vi "Parse Field Type.vi"(6 "Field in":T1={"Name"="", "Number"=0, "Optional"=FALSE, "Repeated"=FALSE, "Type"={"Type"=enum."double", "Subtype"=""}, "Key Type"={"Type"=enum."double", "Subtype"=""}, "Value Type"={"Type"=enum."double", "Subtype"=""}}, 8 "error in (no error)":errorcluster, 10 "Text":string, 11 "ProtoParser in":refnum<class "ProtoParser.lvclass">) -> (0 "error out":errorcluster, 2 "Remaining":string, 3 "ProtoParser out":refnum<class "ProtoParser.lvclass">, 4 "Field":T1={"Name"="", "Number"=0, "Optional"=FALSE, "Repeated"=FALSE, "Type"={"Type"=enum."double", "Subtype"=""}, "Key Type"={"Type"=enum."double", "Subtype"=""}, "Value Type"={"Type"=enum."double", "Subtype"=""}})   [LabVIEW 2024, in "LV-Protoc.lvlib" / "ProtoParser.lvclass"]
uses:
  ProtoParser.lvclass
  ProtoParser.lvclass/ProtoParser.ctl
  LV-Proto/Proto Type.ctl
  LV-Proto/LV-Proto.lvlib
  LV-Proto/Field.ctl
  LV-Proto/Type.ctl
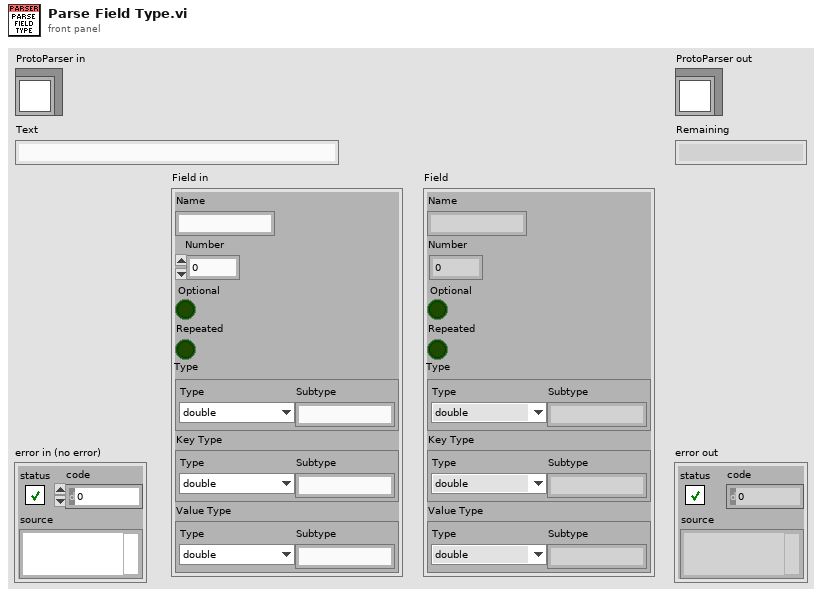
[diagram p1: front panel]
types:
  T1 = typedef "LV-Proto.lvlib/Field.ctl" = cluster{"Name":string, "Number":u32, "Optional":bool, "Repeated":bool, "Type":T2, "Key Type":T2, "Value Type":T2}
  T2 = typedef "LV-Proto.lvlib/Type.ctl" = cluster{"Type":T3, "Subtype":string}
  T3 = typedef "LV-Proto.lvlib/Proto Type.ctl" = enum16{"UNKNOWN", "double", "float", "int32", "int64", "uint32", "uint64", "sint32", "sint64", "fixed32", "fixed64", "sfixed32", "sfixed64", "bool", "string", "bytes", "enum", "map", "message"}
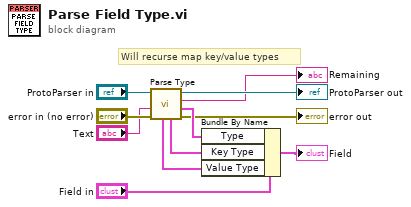
[diagram p0: block diagram]
diagram:
  # "Will recurse map key/value types"
  n1 = call "Parse Type.vi"("error in (no error)"="error in (no error)", "Text"="Text", "ProtoParser in"="ProtoParser in") -> ("error out"=→"error out":errorcluster, "Type"=w7:T2, "Remaining"=→"Remaining":string, "ProtoParser out"=→"ProtoParser out":refnum<class "ProtoParser.lvclass">, "Key Type"=w5:T2, "Value Type"=w6:T2)  [unwired: 3 in]
  n2 = Bundle By Name(cluster="Field in", "Type"=w7, "Key Type"=w5, "Value Type"=w6) -> (→"Field":T1)
